vi "GetControlRefnum.vi"(3 "ErrorIn":errorcluster, 4 "ControlLabelText":string, 5 "VIRefnumIn":refnum<vi>) -> (0 "ErrorOut":errorcluster, 1 "CtlRefnum":refnum<vi>, 2 "VIRefnumThru":refnum<vi>)   [LabVIEW 2023]
doc: "Gets the Refnum for a control or indicator on the FrontPanel, its Clusters or TabControls of a VI by VIRefnumIn.\n\ninfo@becker-hickl.com"
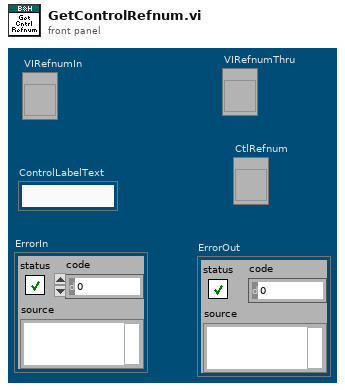
[diagram p1: front panel]
types:
  T1 = enum32{"(CID = 0:  Undefined)", "Application", "VI", "Generic", "Decoration", "Text", "Control", "ColorBox", "Boolean", "RefNum", "LVVariant", "Path", "ListBox", "Table", "Array", "Picture", "ActiveXContainer", "Numeric", "Digital", "NamedNumeric", "ColorRamp", "Slide", "GraphChart", "WaveformChart", "WaveformGraph", "IntensityChart", "IntensityGraph", "String", "IOName", "ComboBox", "Cluster", "Panel", "Knob", "NumericWithScale", "Ring", "Enum", "GObject", "Plot", "Cursor", "NumericText", "Scale", "ColorScale", "GraphScale", "ColorGraphScale", "TypedRefNum", "OldKnobScale", "MulticolumnListbox", "WaveformData", "DSCTag", "DAQChannelName", "VISAResourceName", "IVILogicalName", "SlideScale", "PageSelector", "Page", "TabControl", "ConnectorPane", "DAQmxName", "VIRefNum", "LVObjectRefNum", "AbsTime", "DigitalTable", "TableControl", "MulticolumnListboxControl", "SingleColumnListbox", "SubPanel", "TreeControl", "GenClassTagRef", "GenClassRef", "RotaryColorScale", "PlugInControl", "PlugInDDODummyContainer", "(CID >= 72:  Undefined)"}
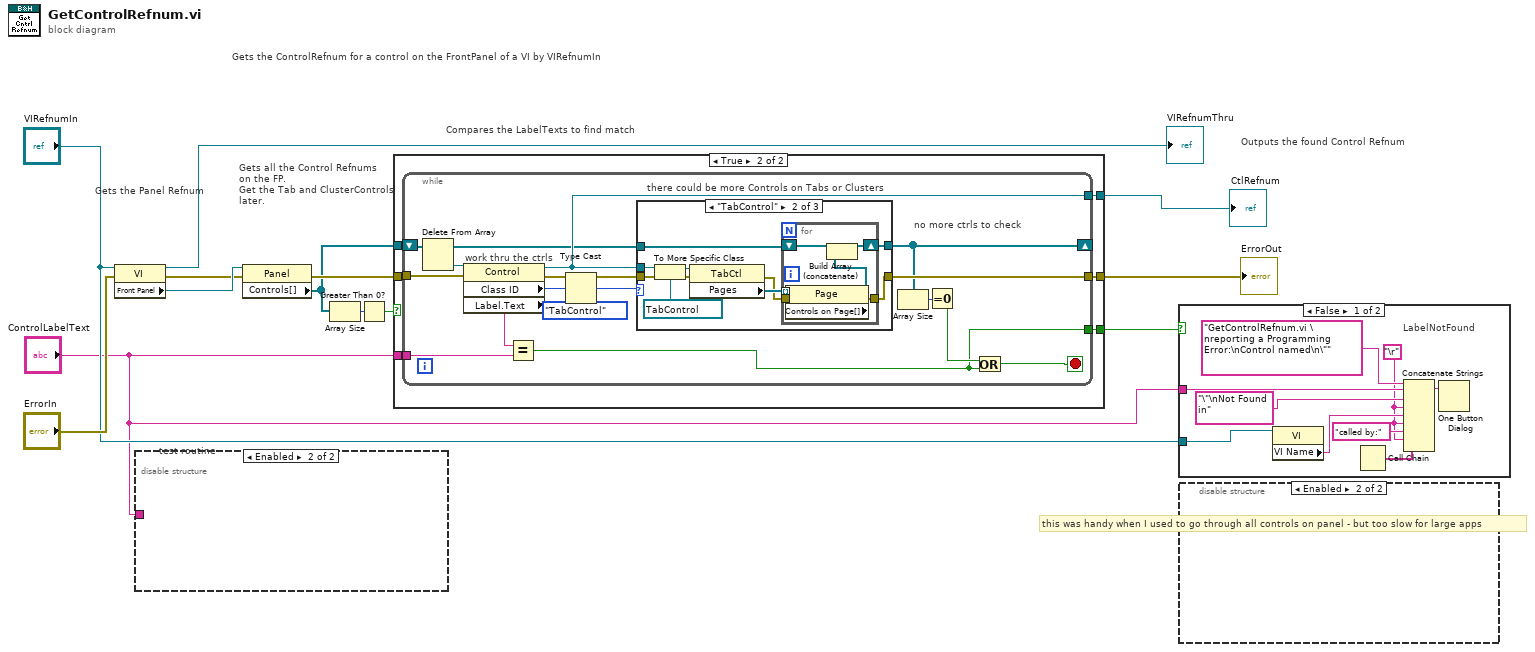
[diagram p0: block diagram]
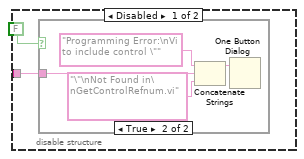
[diagram p2: hidden frame]
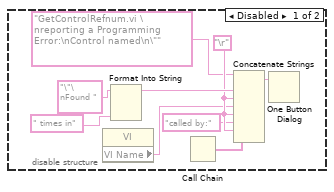
[diagram p4: hidden frame]
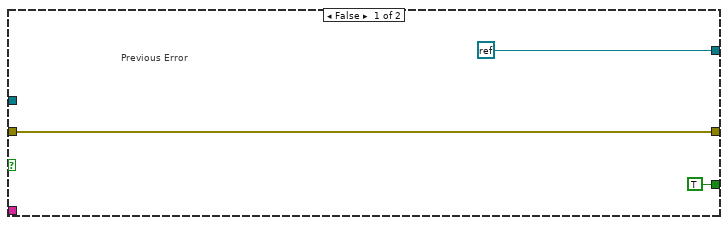
[diagram p6: hidden frame]
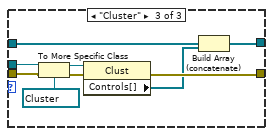
[diagram p8: hidden frame]
diagram:
  # "test routine"
  # "this was handy when I used to go through all controls on panel - but too slow for large apps"
  # "Gets the ControlRefnum for a control on the FrontPanel of a VI by VIRefnumIn"
  # "Outputs the found Control Refnum"
  # "Compares the LabelTexts to find match"
  # "Gets all the Control Refnums\non the FP.\nGet the Tab and ClusterControls\nlater."
  # "Gets the Panel Refnum"
  n1 = property class="VI"(reference="VIRefnumIn", error in="ErrorIn") -> (reference out=→"VIRefnumThru":refnum<vi>, error out=w7:errorcluster, "Front Panel"=w12:refnum<vi>)
  n2 = disable-structure shown="Enabled" {
    disable-tunnel: "ControlLabelText" -> [w14 _]
    frame Disabled {
      n3 = case shown="True" FALSE ("Case Constant\n(See Context Help)") {
        tunnel: w14 -> [_ w16]
        frame False {
        }
        frame True {
          n4 = Concatenate Strings("Programming Error:\nVi to include control \"" ("message"), w16, "\"\nNot Found in\nGetControlRefnum.vi" ("message")) -> (w17:string)
          n5 = One Button Dialog(message=w17) -> ()  [unwired: 2 out]
        }
      }
    }
    frame Enabled {
    }
  }
  n6 = property class="Panel"(reference=w12, error in=w7) -> (error out=w9:errorcluster, "Controls[]"=w6:refnum<vi>[])  [unwired: 1 out]
  n7 = Array Size(array=w6) -> (size(s)=w5:i32)
  n8 = Greater Than 0?(x=w5) -> (x > 0?=w11:bool)
  n9 = case shown="True" w11 {
    tunnel: w9 -> [w22 w28]
    tunnel: [refnum<k0> refnum w27] -> w2
    tunnel: [w22 w26] -> w8
    tunnel: "ControlLabelText" -> [_ w25]
    tunnel: w6 -> [_ w24]
    tunnel: [TRUE w23] -> w1
    frame False {
      # "Previous Error"
    }
    frame True {
      n10 = while {
        tunnel: [w35] -> w27
        tunnel: w28 -> [w45]
        tunnel: [w38] -> w26
        tunnel: w25 -> [w44]
        shift-right: [w32] -> _
        shift-left: w24 -> [w36]
        tunnel: [w29] -> w23
        stop <- w31 stop-if-true
        # "no more ctrls to check"
        # "work thru the ctrls"
        # "there could be more Controls on Tabs or Clusters"
        n11 = Delete From Array "Delete From Array"(array=w36) -> (deleted portion=w37:refnum<vi>, array with subset deleted=w34:refnum<vi>[])  [unwired: 2 in]
        n12 = property class="Control"(reference=w37, error in=w45) -> (reference out=w35:refnum<vi>, error out=w39:errorcluster, "Class ID"=w42:u32, "Label.Text"=w43:string)
        n13 = Equal?(x=w43, y=w44) -> (x = y?=w29:bool)
        n14 = Type Cast(type=T1."TabControl" ("ClassID Name"), x=w42) -> (*(type *) &x=w41:T1)
        n15 = case shown="\"TabControl\"" w41 {
          tunnel: w35 -> [_ w57 w68]
          tunnel: w39 -> [w46 w56 w69]
          tunnel: [w46 w50 w67] -> w38
          tunnel: w34 -> [w47 w49 w66]
          tunnel: [w47 w48 w65] -> w32
          frame "(CID = 0:  Undefined)", Default {
          }
          frame "TabControl" {
            n16 = To More Specific Class(target class=refnum<vi> refnum ("Tab Control"), reference=w57, error in=w56) -> (specific class reference=w54:refnum<vi>, error out=w53:errorcluster)
            n17 = property class="TabCtl"(reference=w54, error in=w53) -> (error out=w51:errorcluster, "Pages"=w52:refnum<vi>[])  [unwired: 1 out]
            n18 = for {
              tunnel: w52 -> [w63] mode=indexing
              tunnel: w51 -> [w62]
              tunnel: [w61] -> w50
              shift-right: [w58] -> w48
              shift-left: w49 -> [w60]
              n19 = property class="Page"(reference=w63, error in=w62) -> (error out=w61:errorcluster, "Controls on Page[]"=w59:refnum<vi>[])  [unwired: 1 out]
              n20 = Build Array (concatenate)(w60, w59) -> (w58:refnum<vi>[])
            }
          }
          frame "Cluster" {
            n21 = To More Specific Class(target class=refnum<vi> refnum ("Tab Control"), reference=w68, error in=w69) -> (specific class reference=w70:refnum<vi>, error out=w72:errorcluster)
            n22 = property class="Clust"(reference=w70, error in=w72) -> (error out=w67:errorcluster, "Controls[]"=w64:refnum<vi>[])  [unwired: 1 out]
            n23 = Build Array (concatenate)(w66, w64) -> (w65:refnum<vi>[])
          }
        }
        n24 = Array Size(array=w32) -> (size(s)=w33:i32)
        n25 = Equal To 0?(x=w33) -> (x = 0?=w30:bool)
        n26 = Or(x=w30, y=w29) -> (x .or. y?=w31:bool)
      }
    }
  }
  "ErrorOut" <- w8
  "CtlRefnum" <- w2
  n27 = case shown="False" w1 {
    tunnel: "ControlLabelText" -> [w76 _]
    tunnel: "VIRefnumIn" -> [w77 _]
    frame False {
      w73 = "\r"
      # "LabelNotFound"
      n28 = property class="VI"(reference=w77) -> ("VI Name"=w78:string)  [unwired: 1 in, 2 out]
      n29 = Call Chain() -> (call chain=w74:string[])
      n30 = Concatenate Strings("GetControlRefnum.vi \nreporting a Programming Error:\nControl named\n\"" ("message"), w76, "\"\nNot Found in" ("message"), w73, w78, w73, "called by:" ("string"), w73, w74) -> (w79:string)
      n31 = One Button Dialog(message=w79) -> ()  [unwired: 2 out]
    }
    frame True {
    }
  }
  n32 = disable-structure shown="Enabled" {
    frame Disabled {
      w90 = "\r"
      # "LabelDouble"
      n33 = property class="VI"() -> (reference=w86:refnum<vi>, "VI Name"=w85:string)  [unwired: 1 in, 2 out]
      n34 = Format Into String(initial string="\"\nFound " ("message"), " times in" ("message")) -> (resulting string=w91:string, w92:bool)  [unwired: 2 in, 1 out]
      n35 = Call Chain() -> (call chain=w89:string[])
      n36 = Concatenate Strings("GetControlRefnum.vi \nreporting a Programming Error:\nControl named\n\"" ("message"), w91, w90, w85, w90, "called by:" ("string"), w90, w89) -> (w84:string, w87:string)
      n37 = One Button Dialog(message=w84) -> ()  [unwired: 2 out]
    }
    frame Enabled {
    }
  }
